vi "Configuration Parse.vi"(8 "error in":errorcluster, 11 "UI Controls":T3={"measurement configuration"={"Automation Test"=FALSE, "Power sequencing file path"="", "RFmxVNA name"="", "vCal Name"="VNA-5633", "RFmxVNA Calset Enable"=FALSE, "RFmxVNA Calset Interpolation"=FALSE, "Calset File Path (String)"="", "RFmxVNA attenuation mode"=enum."s2p File", "RFmxVNA Port1 s2p file path (String)"="", "RFmxVNA Port1 s-parameters orientation"=enum."Port1 Towards DUT", "RFmxVNA Port1 Power Compensation"=FALSE, "RFmxVNA Port2 s2p file path (String)"="", "RFmxVNA Port2 s-parameters orientation"=enum."Port1 Towards DUT", "RFmxVNA Port2 Power Compensation"=FALSE, "Port1 Power Level (dBm)"=0.0, "Port1 Test Receiver Attenuation (dB)"=0.0, "Port2 Power Level (dBm)"=0.0, "Port2 Test Receiver Attenuation (dB)"=0.0, "IF Bandwidth (Hz)"=0.0, "Action"=enum."Calibrate", "Pulse Mode Enabled"=FALSE, "Pulse Period"=0.0, "Pulse Modulator Delay"=0.0, "Pulse Modulator Width"=0.0, "Pulse Acquisition Auto"=FALSE, "Pulse Acquisition Delay"=0.0, "Pulse Acquisition Width"=0.0, "Start Frequency (Hz)"=0.0, "Stop Frequency (Hz)"=0.0, "Number of Points"=0, "Measurement S-Parameters"=[], "Phase Trace Type"=0, "Magnitude Units"=0, "SnP File Path (String)"="", "Averaging Enabled"=FALSE, "Averaging Count"=0}, "measurement results"={"Status"="", "S-Param Name"=[], "S-Param Magnitude"=[], "S-Param Phase"=[], "VNA Status"=""}} {"measurement configuration"."Averaging Count" format="%.0g"; "measurement configuration"."Magnitude Units" items=["dB", "Linear"]; "measurement configuration"."Phase Trace Type" items=["Wrapped", "Unwrapped"]; "measurement configuration"."Stop Frequency (Hz)" format="%.3p"; "measurement configuration"."Start Frequency (Hz)" format="%.3p"; "measurement configuration"."Pulse Acquisition Width" format="%.2p"; "measurement configuration"."Pulse Acquisition Delay" format="%.2p"; "measurement configuration"."Pulse Modulator Width" format="%.2p"; "measurement configuration"."Pulse Modulator Delay" format="%.2p"; "measurement configuration"."Pulse Period" format="%.2p"; "measurement configuration"."IF Bandwidth (Hz)" format="%.2p"; "measurement configuration"."Port2 Test Receiver Attenuation (dB)" format="%.2f"; "measurement configuration"."Port2 Power Level (dBm)" format="%.2f"; "measurement configuration"."Port1 Test Receiver Attenuation (dB)" format="%.2f"; "measurement configuration"."Port1 Power Level (dBm)" format="%.2f"}) -> (0 "error out":errorcluster, 2 "RFmxVNA Settings":T5={"Resource Name"="", "vCal Name"="", "RFmxVNA Calset Enable"=FALSE, "RFmxVNA Calset Interpolation"=FALSE, "Calset File Path"="", "RFmxVNA attenuation mode"=enum."s2p File", "RFmxVNA Port1 s2p file path"="", "RFmxVNA Port1 s-parameters orientation"=enum."Port1 Towards DUT", "RFmxVNA Port1 Power Compensation"=FALSE, "RFmxVNA Port2 s2p file path"="", "RFmxVNA Port2 s-parameters orientation"=enum."Port1 Towards DUT", "RFmxVNA Port2 Power Compensation"=FALSE, "Port1 Power Level (dBm)"=0.0, "Port1 Test Receiver Attenuation (dB)"=0.0, "Port2 Power Level (dBm)"=0.0, "Port2 Test Receiver Attenuation (dB)"=0.0, "IF Bandwidth (Hz)"=0.0, "Frequency Sweep"={"Start Frequency (Hz)"=4000000000.0, "Stop Frequency (Hz)"=26000000000.0, "Number of Points"=200}} {"Frequency Sweep"."Stop Frequency (Hz)" format="%.3p"; "Frequency Sweep"."Start Frequency (Hz)" format="%.3p"; "IF Bandwidth (Hz)" format="%.2p"; "Port2 Test Receiver Attenuation (dB)" format="%.2f"; "Port2 Power Level (dBm)" format="%.2f"; "Port1 Test Receiver Attenuation (dB)" format="%.2f"; "Port1 Power Level (dBm)" format="%.2f"}, 3 "Test Configuration":T4={"Action"=enum."Measure", "Pulse Mode"={"Pulse Mode Enabled"=FALSE, "Pulse Period (s)"=0.0, "Pulse Modulator Delay (s)"=0.0, "Pulse Modulator Width (s)"=0.0, "Pulse Acquisition Auto"=FALSE, "Pulse Acquisition Delay (s)"=0.0, "Pulse Acquisition Width (s)"=0.0}, "Frequency Sweep"={"Start Frequency (Hz)"=0.0, "Stop Frequency (Hz)"=0.0, "Number of Points"=0}, "S-Parameters"=[], "Magnitude Units"=0, "Phase Trace Type"=0, "SnP File Path"="", "Averaging Enabled"=FALSE, "Averaging Count"=0} {"Phase Trace Type" items=["Wrapped", "Unwrapped"]; "Pulse Mode"."Pulse Acquisition Width (s)" format="%.2p"; "Pulse Mode"."Pulse Acquisition Delay (s)" format="%.2p"; "Pulse Mode"."Pulse Modulator Width (s)" format="%.2p"; "Pulse Mode"."Pulse Modulator Delay (s)" format="%.2p"; "Pulse Mode"."Pulse Period (s)" format="%.2p"; "Magnitude Units" items=["dB", "Linear"]; "Frequency Sweep"."Stop Frequency (Hz)" format="%.3p"; "Frequency Sweep"."Start Frequency (Hz)" format="%.3p"})   [LabVIEW 2023, in "FPT_SParam.lvclass"]
uses:
  FPT_SParam.lvclass
  Measurement/Controls/RFmxVNA Config - SParam.ctl
  Measurement/Controls/Test Config - SParam.ctl
  Measurement Configuration.ctl
  Measurement Results.ctl
  FPT_SParam.lvclass/FPT_SParam.ctl
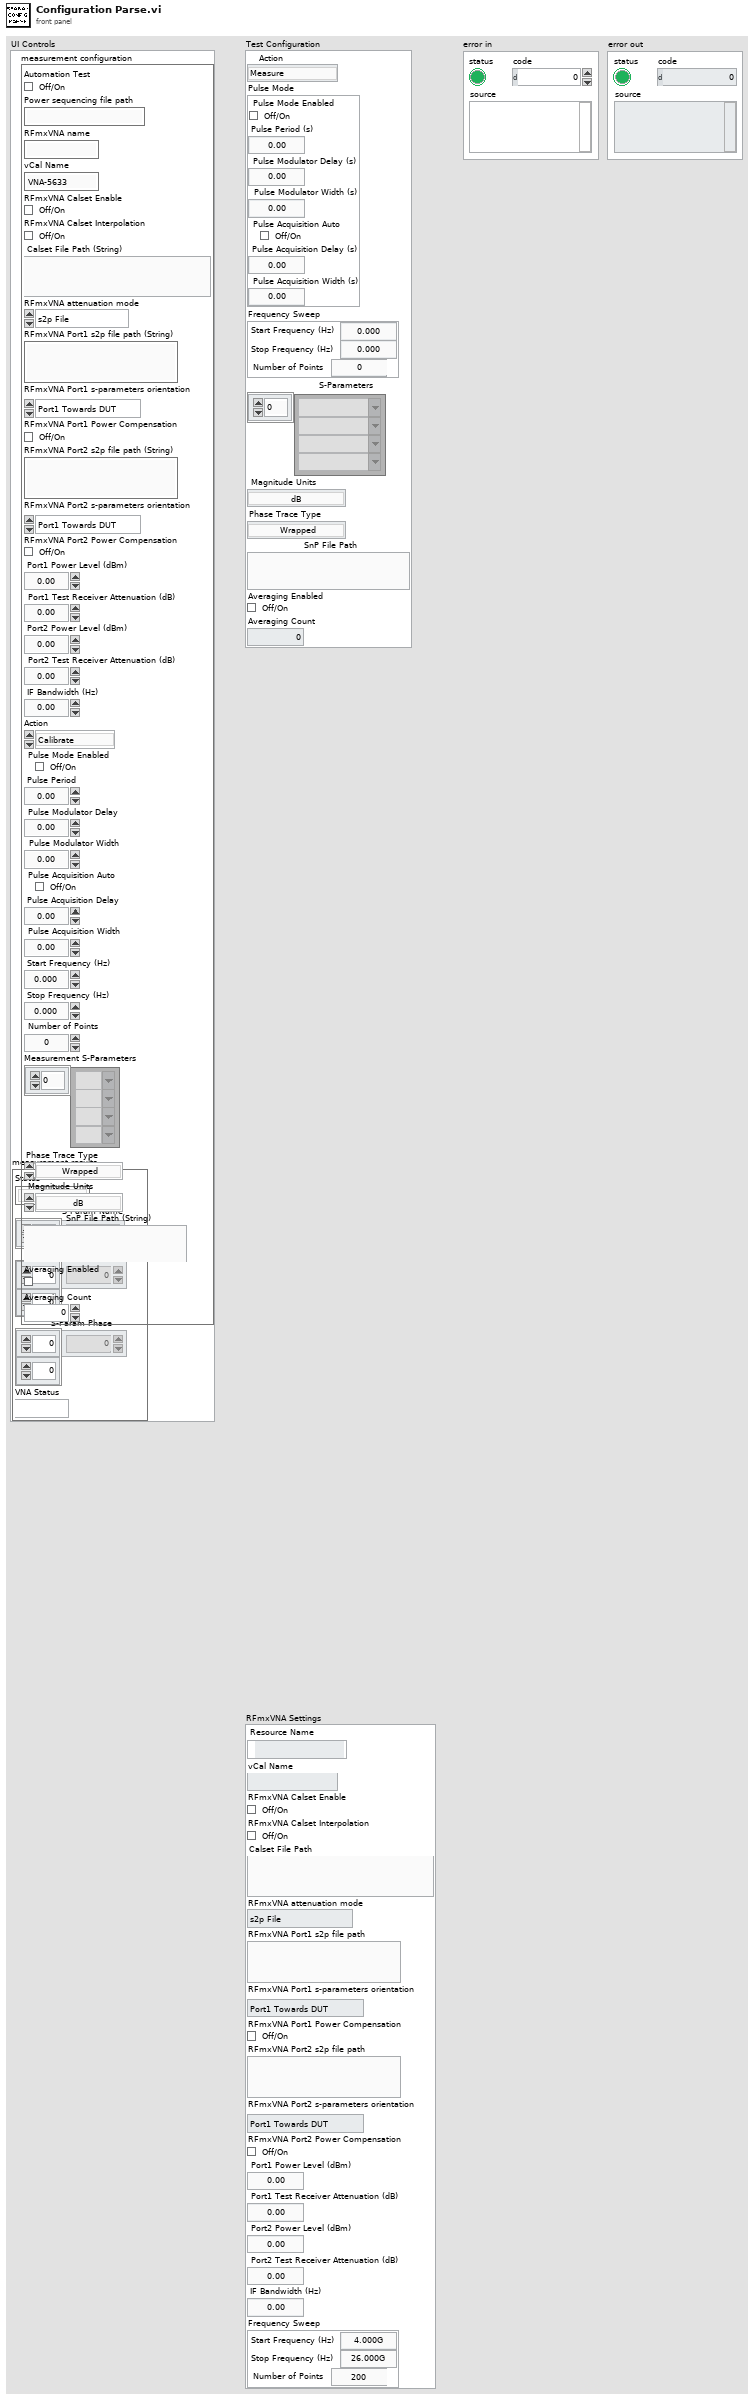
[diagram p1: front panel]
types:
  T1 = typedef "FPT_SParam.lvclass/Measurement Configuration.ctl" = cluster{"Automation Test":bool, "Power sequencing file path":string, "RFmxVNA name":string, "vCal Name":string, "RFmxVNA Calset Enable":bool, "RFmxVNA Calset Interpolation":bool, "Calset File Path (String)":string, "RFmxVNA attenuation mode":enum32{"<None>", "s2p File"}, "RFmxVNA Port1 s2p file path (String)":string, "RFmxVNA Port1 s-parameters orientation":enum32{"Port1 Towards DUT", "Port2 Towards DUT"}, "RFmxVNA Port1 Power Compensation":bool, "RFmxVNA Port2 s2p file path (String)":string, "RFmxVNA Port2 s-parameters orientation":enum32{"Port1 Towards DUT", "Port2 Towards DUT"}, "RFmxVNA Port2 Power Compensation":bool, "Port1 Power Level (dBm)":dbl, "Port1 Test Receiver Attenuation (dB)":dbl, "Port2 Power Level (dBm)":dbl, "Port2 Test Receiver Attenuation (dB)":dbl, "IF Bandwidth (Hz)":dbl, "Action":enum32{"Calibrate", "Measure"}, "Pulse Mode Enabled":bool, "Pulse Period":dbl, "Pulse Modulator Delay":dbl, "Pulse Modulator Width":dbl, "Pulse Acquisition Auto":bool, "Pulse Acquisition Delay":dbl, "Pulse Acquisition Width":dbl, "Start Frequency (Hz)":dbl, "Stop Frequency (Hz)":dbl, "Number of Points":i32, "Measurement S-Parameters":string[], "Phase Trace Type":i32, "Magnitude Units":i32, "SnP File Path (String)":string, "Averaging Enabled":bool, "Averaging Count":u32}
  T2 = typedef "FPT_SParam.lvclass/Measurement Results.ctl" = cluster{"Status":string, "S-Param Name":string[], "S-Param Magnitude":dbl[][], "S-Param Phase":dbl[][], "VNA Status":string}
  T3 = cluster{"measurement configuration":T1, "measurement results":T2}
  T4 = typedef "Test Config - SParam.ctl" = cluster{"Action":enum16{"Calibrate", "Measure"}, "Pulse Mode":cluster{"Pulse Mode Enabled":bool, "Pulse Period (s)":dbl, "Pulse Modulator Delay (s)":dbl, "Pulse Modulator Width (s)":dbl, "Pulse Acquisition Auto":bool, "Pulse Acquisition Delay (s)":dbl, "Pulse Acquisition Width (s)":dbl}, "Frequency Sweep":cluster{"Start Frequency (Hz)":dbl, "Stop Frequency (Hz)":dbl, "Number of Points":i32}, "S-Parameters":string[], "Magnitude Units":i32, "Phase Trace Type":i32, "SnP File Path":string, "Averaging Enabled":bool, "Averaging Count":u32}
  T5 = typedef "RFmxVNA Config - SParam.ctl" = cluster{"Resource Name":refnum<k15>, "vCal Name":string, "RFmxVNA Calset Enable":bool, "RFmxVNA Calset Interpolation":bool, "Calset File Path":string, "RFmxVNA attenuation mode":enum32{"<None>", "s2p File"}, "RFmxVNA Port1 s2p file path":string, "RFmxVNA Port1 s-parameters orientation":enum32{"Port1 Towards DUT", "Port2 Towards DUT"}, "RFmxVNA Port1 Power Compensation":bool, "RFmxVNA Port2 s2p file path":string, "RFmxVNA Port2 s-parameters orientation":enum32{"Port1 Towards DUT", "Port2 Towards DUT"}, "RFmxVNA Port2 Power Compensation":bool, "Port1 Power Level (dBm)":dbl, "Port1 Test Receiver Attenuation (dB)":dbl, "Port2 Power Level (dBm)":dbl, "Port2 Test Receiver Attenuation (dB)":dbl, "IF Bandwidth (Hz)":dbl, "Frequency Sweep":cluster{"Start Frequency (Hz)":dbl, "Stop Frequency (Hz)":dbl, "Number of Points":i32}}
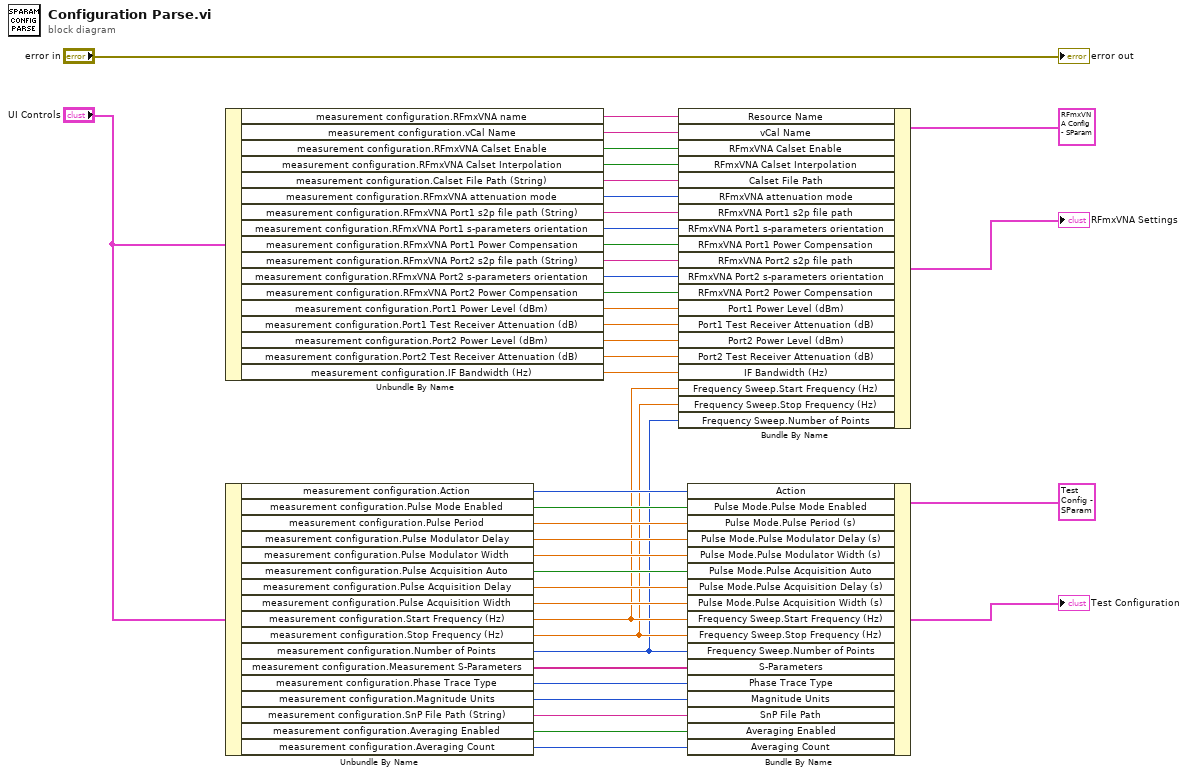
[diagram p0: block diagram]
diagram:
  n1 = Unbundle By Name("UI Controls") -> ("measurement configuration.RFmxVNA name"=w36:string, "measurement configuration.vCal Name"=w3:string, "measurement configuration.RFmxVNA Calset Enable"=w5:bool, "measurement configuration.RFmxVNA Calset Interpolation"=w4:bool, "measurement configuration.Calset File Path (String)"=w35:string, "measurement configuration.RFmxVNA attenuation mode"=w9:enum32{"<None>", "s2p File"}, "measurement configuration.RFmxVNA Port1 s2p file path (String)"=w16:string, "measurement configuration.RFmxVNA Port1 s-parameters orientation"=w15:enum32{"Port1 Towards DUT", "Port2 Towards DUT"}, "measurement configuration.RFmxVNA Port1 Power Compensation"=w10:bool, "measurement configuration.RFmxVNA Port2 s2p file path (String)"=w13:string, "measurement configuration.RFmxVNA Port2 s-parameters orientation"=w12:enum32{"Port1 Towards DUT", "Port2 Towards DUT"}, "measurement configuration.RFmxVNA Port2 Power Compensation"=w11:bool, "measurement configuration.Port1 Power Level (dBm)"=w34:dbl, "measurement configuration.Port1 Test Receiver Attenuation (dB)"=w33:dbl, "measurement configuration.Port2 Power Level (dBm)"=w32:dbl, "measurement configuration.Port2 Test Receiver Attenuation (dB)"=w31:dbl, "measurement configuration.IF Bandwidth (Hz)"=w30:dbl)
  n2 = Unbundle By Name("UI Controls") -> ("measurement configuration.Action"=w28:enum32{"Calibrate", "Measure"}, "measurement configuration.Pulse Mode Enabled"=w27:bool, "measurement configuration.Pulse Period"=w26:dbl, "measurement configuration.Pulse Modulator Delay"=w25:dbl, "measurement configuration.Pulse Modulator Width"=w24:dbl, "measurement configuration.Pulse Acquisition Auto"=w23:bool, "measurement configuration.Pulse Acquisition Delay"=w22:dbl, "measurement configuration.Pulse Acquisition Width"=w21:dbl, "measurement configuration.Start Frequency (Hz)"=w8:dbl, "measurement configuration.Stop Frequency (Hz)"=w7:dbl, "measurement configuration.Number of Points"=w6:i32, "measurement configuration.Measurement S-Parameters"=w14:string[], "measurement configuration.Phase Trace Type"=w20:i32, "measurement configuration.Magnitude Units"=w19:i32, "measurement configuration.SnP File Path (String)"=w18:string, "measurement configuration.Averaging Enabled"=w2:bool, "measurement configuration.Averaging Count"=w1:u32)
  n3 = Bundle By Name(cluster=T5 {"Resource Name"="VNA-5633", "vCal Name"="", "RFmxVNA Calset Enable"=FALSE, "RFmxVNA Calset Interpolation"=FALSE, "Calset File Path"="", "RFmxVNA attenuation mode"=enum."s2p File", "RFmxVNA Port1 s2p file path"="", "RFmxVNA Port1 s-parameters orientation"=enum."Port1 Towards DUT", "RFmxVNA Port1 Power Compensation"=FALSE, "RFmxVNA Port2 s2p file path"="", "RFmxVNA Port2 s-parameters orientation"=enum."Port1 Towards DUT", "RFmxVNA Port2 Power Compensation"=FALSE, "Port1 Power Level (dBm)"=-10.0, "Port1 Test Receiver Attenuation (dB)"=0.0, "Port2 Power Level (dBm)"=-10.0, "Port2 Test Receiver Attenuation (dB)"=0.0, "IF Bandwidth (Hz)"=100000.0, "Frequency Sweep"={"Start Frequency (Hz)"=4000000000.0, "Stop Frequency (Hz)"=26000000000.0, "Number of Points"=200}} ("RFmxVNA Settings"), "Resource Name"=w36, "vCal Name"=w3, "RFmxVNA Calset Enable"=w5, "RFmxVNA Calset Interpolation"=w4, "Calset File Path"=w35, "RFmxVNA attenuation mode"=w9, "RFmxVNA Port1 s2p file path"=w16, "RFmxVNA Port1 s-parameters orientation"=w15, "RFmxVNA Port1 Power Compensation"=w10, "RFmxVNA Port2 s2p file path"=w13, "RFmxVNA Port2 s-parameters orientation"=w12, "RFmxVNA Port2 Power Compensation"=w11, "Port1 Power Level (dBm)"=w34, "Port1 Test Receiver Attenuation (dB)"=w33, "Port2 Power Level (dBm)"=w32, "Port2 Test Receiver Attenuation (dB)"=w31, "IF Bandwidth (Hz)"=w30, "Frequency Sweep.Start Frequency (Hz)"=w8, "Frequency Sweep.Stop Frequency (Hz)"=w7, "Frequency Sweep.Number of Points"=w6) -> (→"RFmxVNA Settings":T5)
  n4 = Bundle By Name(cluster=T4 {"Action"=enum."Measure", "Pulse Mode"={"Pulse Mode Enabled"=FALSE, "Pulse Period (s)"=0.001, "Pulse Modulator Delay (s)"=0.0, "Pulse Modulator Width (s)"=0.0001, "Pulse Acquisition Auto"=FALSE, "Pulse Acquisition Delay (s)"=2e-05, "Pulse Acquisition Width (s)"=4.665e-05}, "Frequency Sweep"={"Start Frequency (Hz)"=4000000000.0, "Stop Frequency (Hz)"=26000000000.0, "Number of Points"=200}, "S-Parameters"=["S11", "S12", "S21", "S22"], "Magnitude Units"=0, "Phase Trace Type"=0, "SnP File Path"="", "Averaging Enabled"=FALSE, "Averaging Count"=0} ("Test Configuration"), "Action"=w28, "Pulse Mode.Pulse Mode Enabled"=w27, "Pulse Mode.Pulse Period (s)"=w26, "Pulse Mode.Pulse Modulator Delay (s)"=w25, "Pulse Mode.Pulse Modulator Width (s)"=w24, "Pulse Mode.Pulse Acquisition Auto"=w23, "Pulse Mode.Pulse Acquisition Delay (s)"=w22, "Pulse Mode.Pulse Acquisition Width (s)"=w21, "Frequency Sweep.Start Frequency (Hz)"=w8, "Frequency Sweep.Stop Frequency (Hz)"=w7, "Frequency Sweep.Number of Points"=w6, "S-Parameters"=w14, "Phase Trace Type"=w20, "Magnitude Units"=w19, "SnP File Path"=w18, "Averaging Enabled"=w2, "Averaging Count"=w1) -> (→"Test Configuration":T4)
  "error out" <- "error in"
